vi "Start Timer.vi"(8 "error in (no error)":errorcluster, 10 "Time Target (s)":i32, 11 "Timer in":refnum<class "Timer.lvclass">) -> (0 "error out":errorcluster, 3 "Timer out":refnum<class "Timer.lvclass">)   [LabVIEW 2019, in "Timer.lvlib" / "Timer.lvclass"]
uses:
  Timer.lvclass
  Timer.lvclass/Timer.ctl
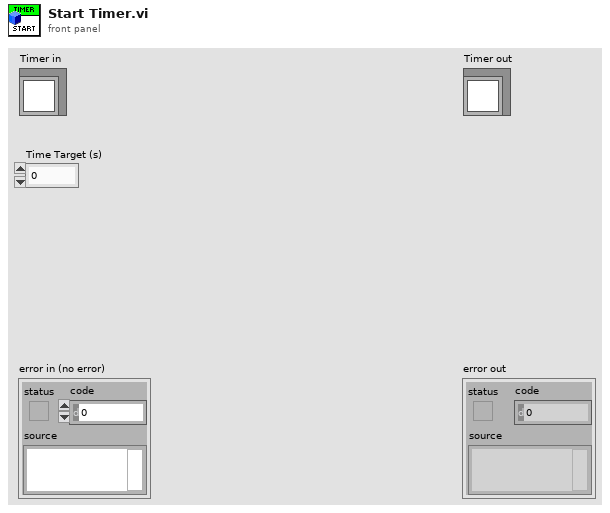
[diagram p1: front panel]
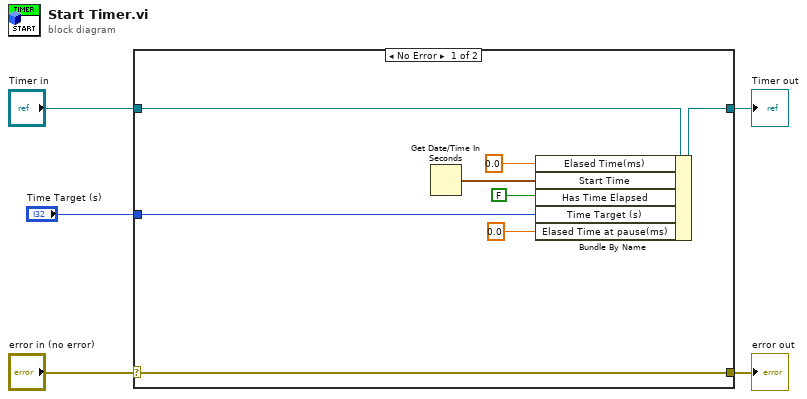
[diagram p0: block diagram]
diagram:
  n1 = case shown="No Error" "error in (no error)" {
    selector: "error in (no error)" -> [w13 w15]
    tunnel: [w13 w15] -> w4
    tunnel: [w11 w14] -> w2
    tunnel: "Timer in" -> [w12 w14]
    tunnel: "Time Target (s)" -> [w8 _]
    frame No Error {
      n2 = Get Date/Time In Seconds() -> (seconds since 1Jan1904=w10:timestamp)
      n3 = Bundle By Name(cluster=w12, "Elased Time(ms)"=0.0, "Start Time"=w10, "Has Time Elapsed"=FALSE, "Time Target (s)"=w8, "Elased Time at pause(ms)"=0.0) -> (w11:refnum<class "Timer.lvclass">)
    }
    frame Error {
    }
  }
  "error out" <- w4
  "Timer out" <- w2
